vi "RFmx_An_SFDR_Disp.vi"(8 "Int_Bandwidth(Hz)":dbl=1000000.0 format="%#_6p", 9 "Signal_Bandwidth(Hz)":dbl=20000000.0 format="%#_6p", 11 "IMD_Spectrum_in":cluster{"x0":dbl, "dx":dbl, "y":sgl[]}={"x0"=989999984.4503028, "dx"=999.4019138756557, "y"=array[20012 elements]}) -> (2 "PeakPwrs_Data":sgl[](array[numeric])=[750000.0, -20.734814, 53.66733, 3.5194657] format="%#_6p", 3 "IMD_Spectrum_Out":cluster{"x0":dbl, "dx":dbl, "y":sgl[]}[](array[cluster])=[{"x0"=989999984.4503028, "dx"=999.4019138756557, "y"=array[20012 elements]}, {"x0"=989999984.4503028, "dx"=999.4019138756557, "y"=array[20012 elements]}])   [LabVIEW 2014]
panel:
  out "size(s)":i32
  out "SFDR_Spectrum":cluster{"x0":dbl, "dx":dbl, "y":sgl[]}[](graph)
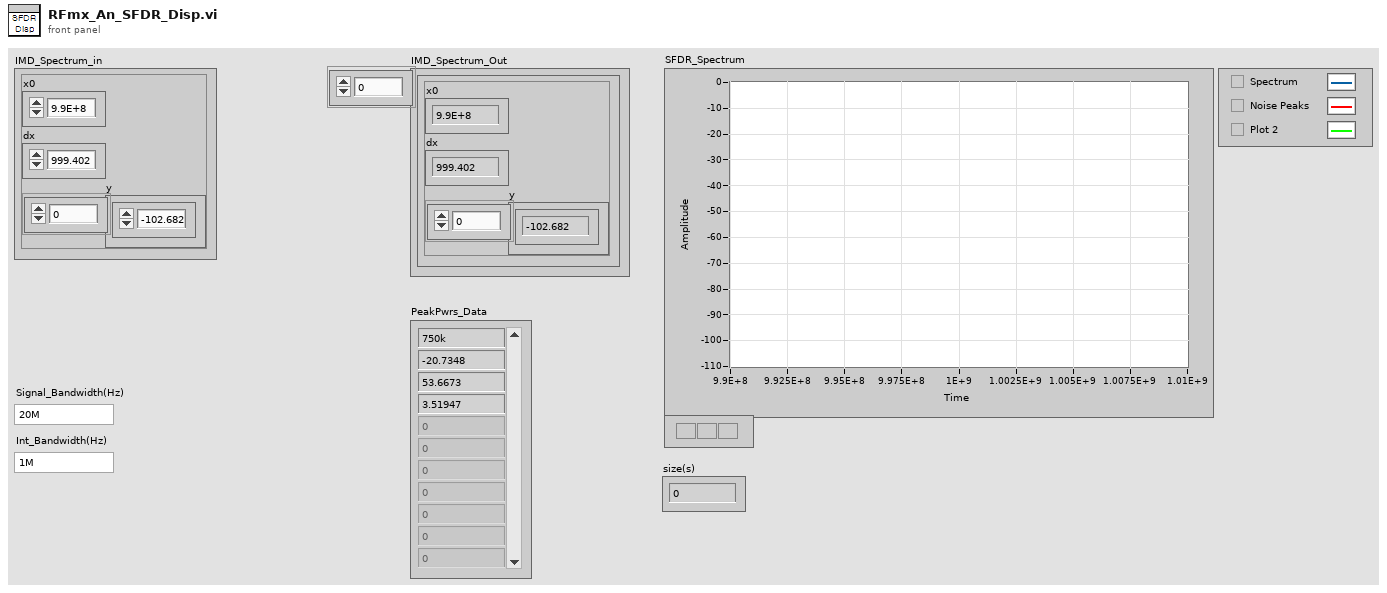
[diagram p1: front panel]
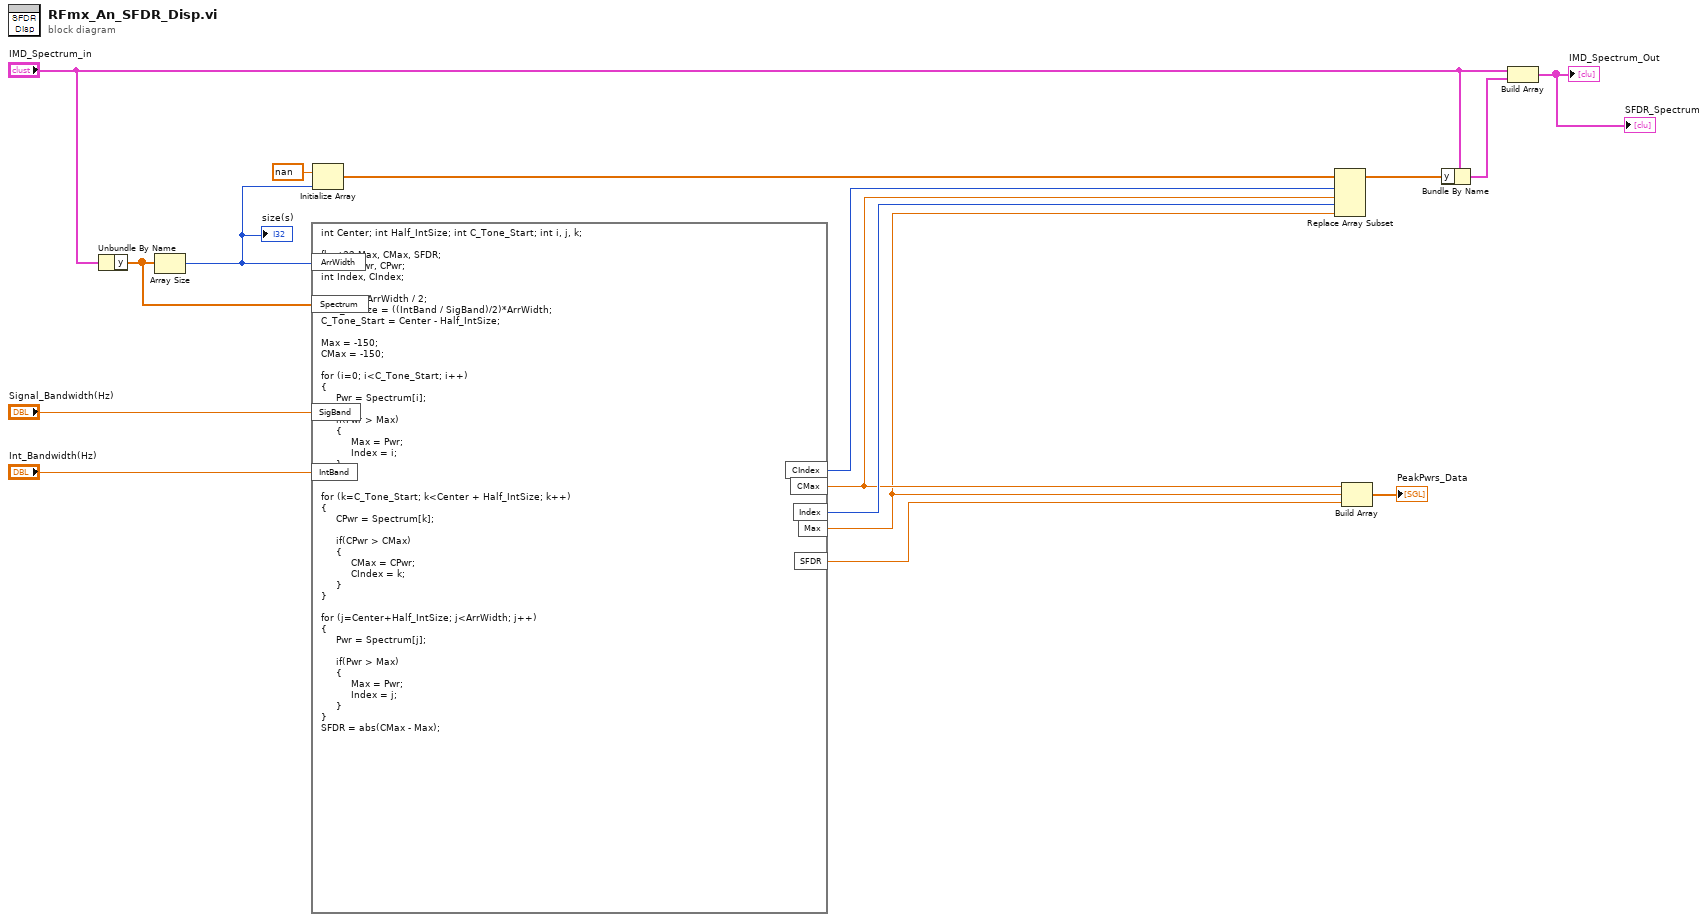
[diagram p0: block diagram]
diagram:
  n1 = Unbundle By Name("IMD_Spectrum_in") -> ("y"=w10:sgl[])
  n2 = Array Size(array=w10) -> (size(s)=w14:i32)
  "size(s)" <- w14
  n3 = formula code="int Center; int Half_IntSize; int C_Tone_Start; int i, j, k;\n\nfloat32 Max, CMax, SFDR;\nfloat32 Pwr, CPwr;\nint Index, CIndex;\n\nCenter = ArrWidth / 2;\nHalf_IntSize = ((IntBand / SigBand)/2)*ArrWidth;\nC_Tone_Start = Center - Half_IntSize;\n\nMax = -150;\nCMax = -150;\n\nfor (i=0; i<C_Tone_Start; i++)\n{\n     Pwr = Spectrum[i];\n\n     if(Pwr > Max)\n     {\n          Max = Pwr;\n          Index = i;\n     }\n}\n\nfor (k=C_Tone_Start; k<Center + Half_IntSize; k++)\n{\n     CPwr = Spectrum[k];\n\n     if(CPwr > CMax)\n     {\n          CMax = CPwr;\n          CIndex = k;\n     }     \n}\n\nfor (j=Center+Half_IntSize; j<ArrWidth; j++)\n{\n     Pwr = Spectrum[j];\n\n     if(Pwr > Max)\n     {\n          Max = Pwr;\n          Index = j;\n     }\n}\nSFDR = abs(CMax - Max);"("SigBand"="Signal_Bandwidth(Hz)", "IntBand"="Int_Bandwidth(Hz)", "ArrWidth"=w14, "Spectrum"=w10) -> ("Max"=w3:sgl, "Index"=w5:i32, "SFDR"=w1:sgl, "CIndex"=w6:i32, "CMax"=w4:sgl)
  n4 = Initialize Array(sgl nan ("element"), w14) -> (w12:sgl[])
  n5 = Replace Array Subset(array=w12, new element #1=w4, index #1=w6, new element #2=w3, index #2=w5) -> (w8:sgl[])
  n6 = Build Array(w4, w3, w1) -> (→"PeakPwrs_Data":sgl[])
  n7 = Bundle By Name(cluster="IMD_Spectrum_in", "y"=w8) -> (w11:cluster{"x0":dbl, "dx":dbl, "y":sgl[]})
  n8 = Build Array("IMD_Spectrum_in", w11) -> (→"IMD_Spectrum_Out" →"SFDR_Spectrum":cluster{"x0":dbl, "dx":dbl, "y":sgl[]}[])
